vi "Motor_Lumicks_Meng.vi"() -> ()   [LabVIEW 2014]
uses:
  <vilib>/userdefined/High Color/IMAQdx.ctl
  <vilib>/Utility/inputDevices.llb/joystickAcquire.vi
  <vilib>/Utility/inputDevices.llb/closeJoystick.vi
  <vilib>/vision/driver/NI_Vision_Acquisition_Software.lvlib
panel:
  out "error out 2":errorcluster
  out "Image":T1(plugin-control)
  in  "Goto Channel 5":bool
  in  "Goto Channel 4":bool
  in  "Capture Channel 5":bool
  in  "Capture Channel 4":bool
  out "Channel 5":T2={"X Pos (mm)"=0.00014575559, "Y Pos (mm)"=-0.0013701026, "Z Pos (mm)"=0.004635028} {"Y Pos (mm)" format="%.3f"; "Z Pos (mm)" format="%.3f"; "X Pos (mm)" format="%.3f"}
  out "Channel 4":T2={"X Pos (mm)"=0.00014575559, "Y Pos (mm)"=-0.0013701026, "Z Pos (mm)"=0.004635028} {"Y Pos (mm)" format="%.3f"; "Z Pos (mm)" format="%.3f"; "X Pos (mm)" format="%.3f"}
  in  "Stop All":bool=TRUE
  out "button 4":bool
  in  "button 3":bool
  in  "Motor Cruise Param":T3={"X Acc (mm/s^2)"=0.1, "X Vmax (mm/s)"=1.0, "Y Acc (mm/s^2)"=0.3, "Y Vmax (mm/s)"=1.0, "Z Acc (mm/s^2)"=0.1, "Z Vmax (mm/s)"=0.1}
  out "XYZ position":sgl[](array[numeric])=[1.7793261, 1.7925023, 3.857043]
  in  "Motor Limits":T4={"XMAX"=12.0, "XMIN"=-12.0, "YMAX"=12.0, "YMIN"=-12.0, "ZMAX"=10.0, "ZMIN"=-10.0}
  in  "Motor settings (X,Y)":cluster{"Vmax (mm/s)":sgl, "Acc (mm/s/s)":sgl}={"Vmax (mm/s)"=0.05, "Acc (mm/s/s)"=0.2}
  in  "Motor settings (Z)":cluster{"Vmax (mm/s)":sgl, "Acc (mm/s/s)":sgl}={"Vmax (mm/s)"=0.02, "Acc (mm/s/s)"=0.2}
  in  "Capture Channel 3":bool
  in  "Capture Channel 2":bool
  in  "Capture Channel 1":bool
  in  "Goto Channel 2":bool
  in  "Goto Channel 3":bool
  in  "Goto Channel 1":bool
  out "Channel 1":T2={"X Pos (mm)"=2.683244, "Y Pos (mm)"=-0.037109375, "Z Pos (mm)"=0.2016383} {"Y Pos (mm)" format="%.3f"; "Z Pos (mm)" format="%.3f"; "X Pos (mm)" format="%.3f"}
  out "Channel 2":T2={"X Pos (mm)"=2.3714144, "Y Pos (mm)"=-0.4775245, "Z Pos (mm)"=0.20615672} {"Y Pos (mm)" format="%.3f"; "Z Pos (mm)" format="%.3f"; "X Pos (mm)" format="%.3f"}
  out "Channel 3":T2={"X Pos (mm)"=3.6928055, "Y Pos (mm)"=-0.788188, "Z Pos (mm)"=0.19962686} {"Y Pos (mm)" format="%.3f"; "Z Pos (mm)" format="%.3f"; "X Pos (mm)" format="%.3f"}
  out "error out":errorcluster
  in  "MG17Motor Z":refnum<k7>(container)
  in  "MG17Motor Y":refnum<k7>(container)
  in  "MG17Motor X":refnum<k7>(container)
  out "Stage Moving":bool
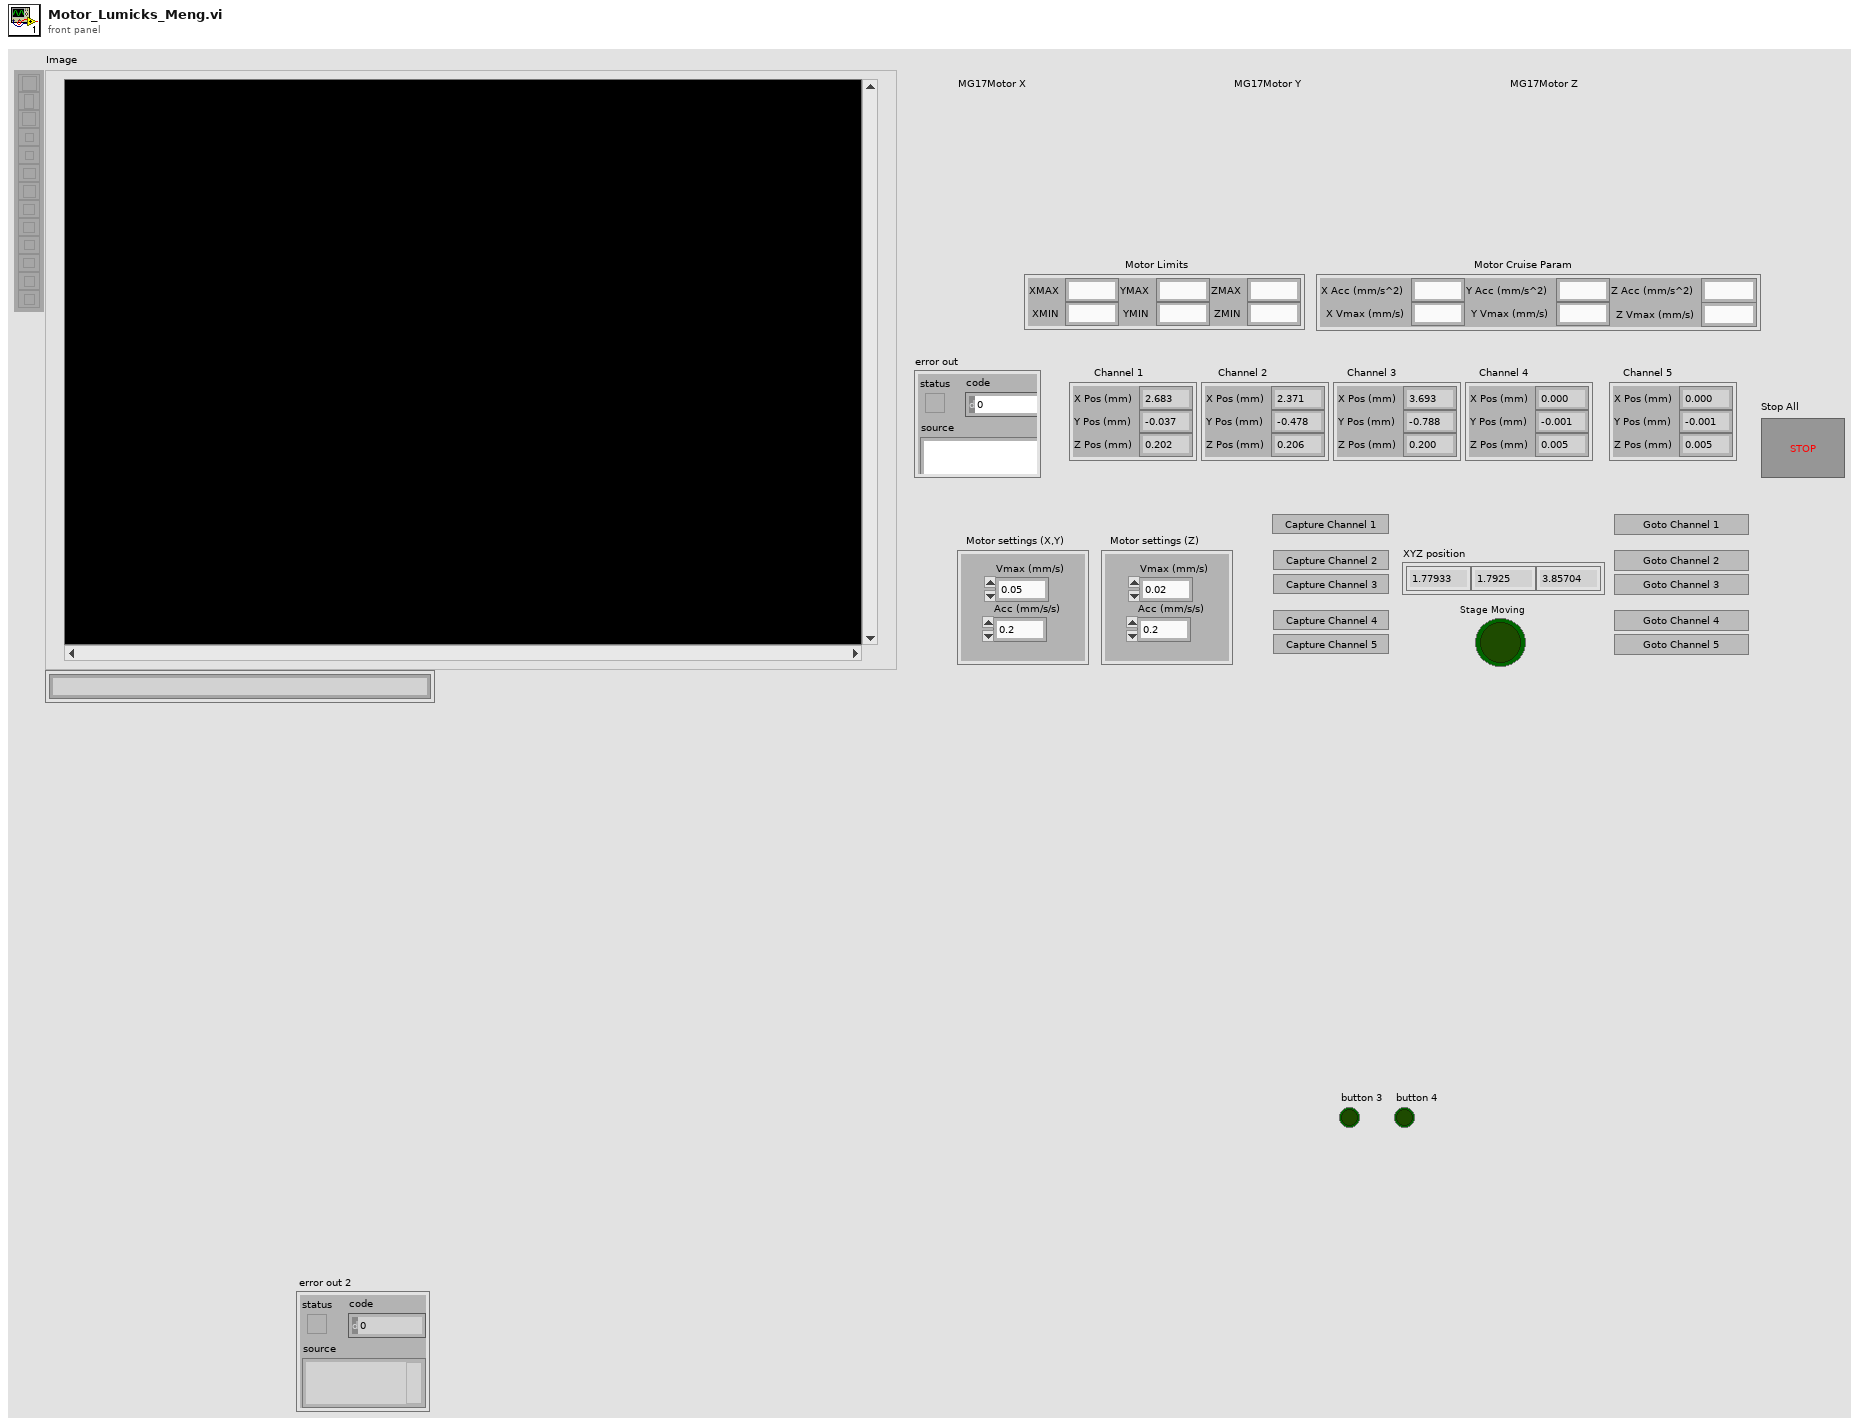
[diagram p1: front panel]
types:
  T1 = typedef "IMAQ Image.ctl" = refnum<image>
  T2 = cluster{"X Pos (mm)":sgl, "Y Pos (mm)":sgl, "Z Pos (mm)":sgl}
  T3 = cluster{"X Acc (mm/s^2)":sgl, "X Vmax (mm/s)":sgl, "Y Acc (mm/s^2)":sgl, "Y Vmax (mm/s)":sgl, "Z Acc (mm/s^2)":sgl, "Z Vmax (mm/s)":sgl}
  T4 = cluster{"XMAX":sgl, "XMIN":sgl, "YMAX":sgl, "YMIN":sgl, "ZMAX":sgl, "ZMIN":sgl}
  T5 = typedef "IMAQdx.ctl" = refnum<k21>
  T6 = typedef "Image Type" = u32
  T7 = cluster{"X axis":i32, "Y axis":i32, "Z axis":i32, "X axis rotation":i32, "Y axis rotation":i32, "Z axis rotation":i32, "U axis":i32, "V axis":i32}
  T8 = cluster{"button 1":bool, "button 2":bool, "button 3":bool, "button 4":bool, "button 5":bool, "button 6":bool, "button 7":bool, "button 8":bool, "button 9":bool, "button 10":bool, "button 11":bool, "button 12":bool, "button 13":bool, "button 14":bool, "button 15":bool, "button 16":bool, "button 17":bool, "button 18":bool, "button 19":bool, "button 20":bool, "button 21":bool, "button 22":bool, "button 23":bool, "button 24":bool, "button 25":bool, "button 26":bool, "button 27":bool, "button 28":bool, "button 29":bool, "button 30":bool, "button 31":bool, "button 32":bool}
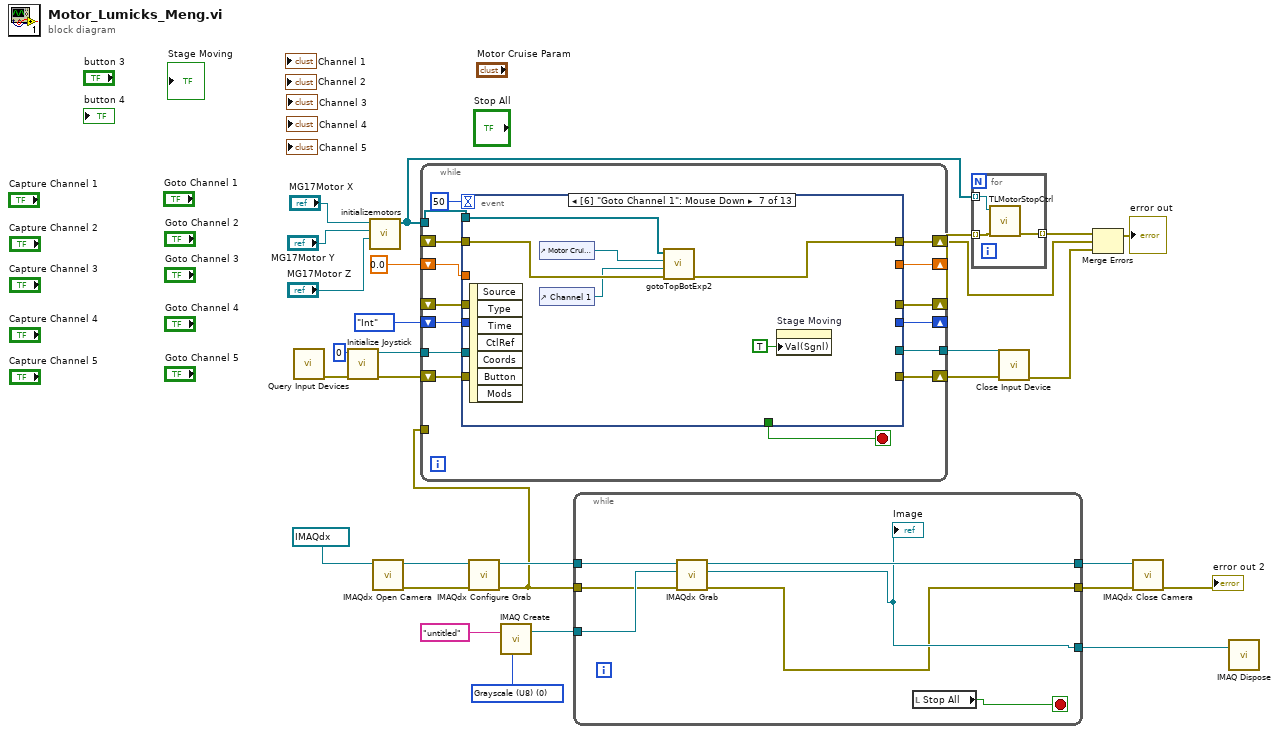
[diagram p0: block diagram]
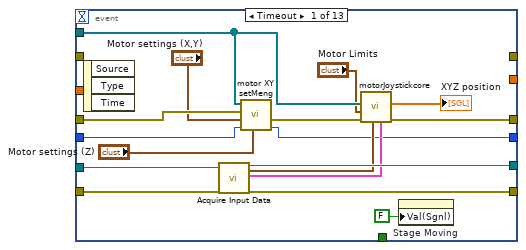
[diagram p2: hidden frame]
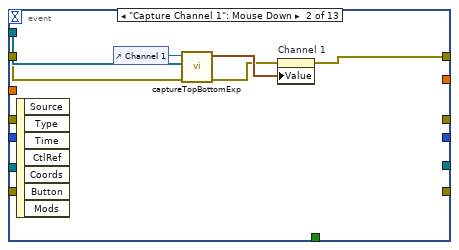
[diagram p3: hidden frame]
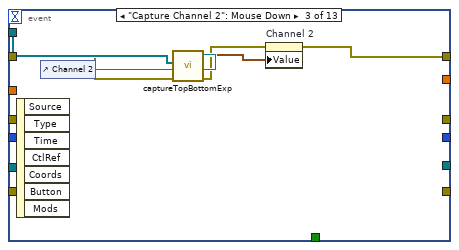
[diagram p4: hidden frame]
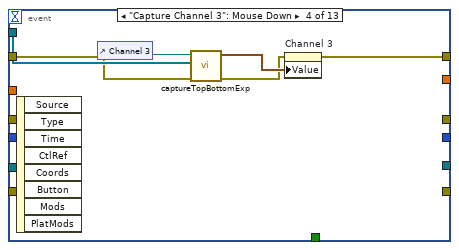
[diagram p5: hidden frame]
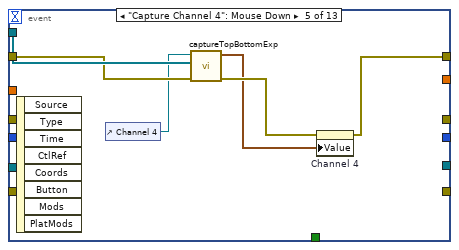
[diagram p6: hidden frame]
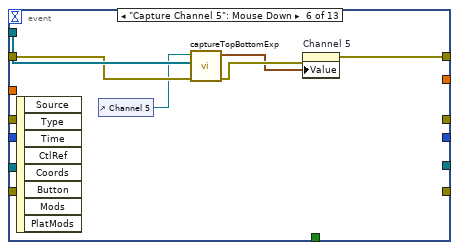
[diagram p7: hidden frame]
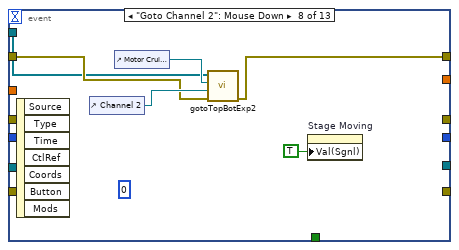
[diagram p8: hidden frame]
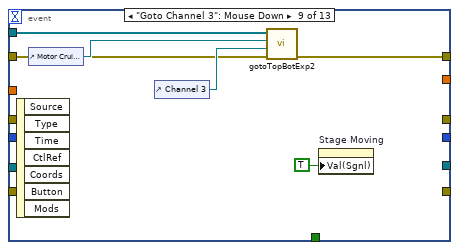
[diagram p9: hidden frame]
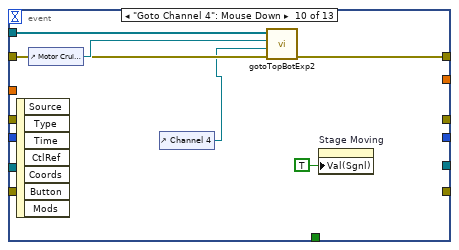
[diagram p10: hidden frame]
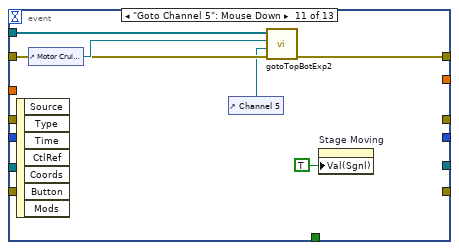
[diagram p11: hidden frame]
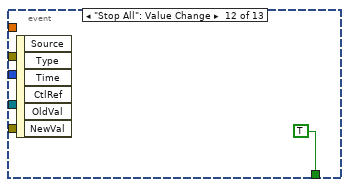
[diagram p12: hidden frame]
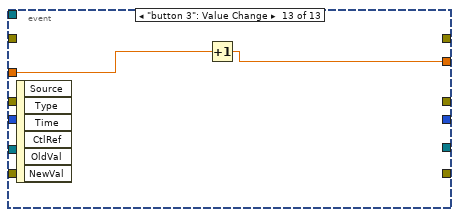
[diagram p13: hidden frame]
diagram:
  w6 = T6 0 items=["Grayscale (U8)", "Grayscale (I16)", "Grayscale (SGL)", "Complex (CSG)", "RGB (U32)", "HSL (U32)", "RGB (U64)", "Grayscale (U16)"] ("Image Type")
  n1 = call <vilib>:"Query Input Devices.vi"() -> ("error out"=w22:errorcluster)  [unwired: 8 in, 3 out]
  n2 = call <vilib>:"Initialize Joystick.vi"("error in (no error)"=w22, "device index"=0) -> ("error out"=w19:errorcluster, "device ID"=w20:refnum<k1>)  [unwired: 8 in]
  n3 = call "initializemotors.vi"("MG17Motor Z"="MG17Motor Z", "MG17Motor Y"="MG17Motor Y", "Automation Refnum in"="MG17Motor X") -> ("Array 2"=w24:refnum<k7>[])  [unwired: 7 in, 1 out]
  n4 = call <vilib>:"IMAQdx Open Camera.vi"("Session In"=T5 "cam0") -> ("error out"=w10:errorcluster, "Session Out"=w9:T5)  [unwired: 9 in]
  n5 = call <vilib>:"IMAQdx Configure Grab.vi"("error in"=w10, "Session In"=w9) -> ("error out"=w1:errorcluster, "Session Out"=w8:T5)  [unwired: 8 in]
  n6 = while {
    tunnel: w24 -> [w44]
    shift-right: [w43] -> w14
    shift-left: _ -> [w42]
    shift-right: [w39] -> _
    shift-left: 0.0 -> [w40]
    tunnel: w20 -> [w38]
    shift-right: [w36] -> w18
    shift-left: w19 -> [w37]
    tunnel: [w35] -> w17
    shift-right: [w34] -> w15
    shift-left: _ -> [w33]
    shift-right: [w31] -> _
    shift-left: enum16{"Int", "Set"}."Int" ("Enum") -> [w32]
    tunnel: w1 -> [_]
    stop <- w41 stop-if-true
    n7 = event shown="[6] \"Goto Channel 1\": Mouse Down" {
      selector: _ -> [_ _ _ _ _ _ _ _ _ _ _ _ _]
      dyn-events: _ -> [_ _ _ _ _ _ _ _ _ _ _ _ _]
      timeout: 50 -> [_ _ _ _ _ _ _ _ _ _ _ _ _]
      tunnel: w44 -> [w51 w67 w72 w79 w85 w91 w93 w99 w105 w112 w118 _ _]
      tunnel: [_ w64 w68 w74 w81 w86 w96 w100 w106 w113 w119 _ _] -> w43
      tunnel: w42 -> [_ w63 w71 w77 w84 w90 w97 w101 w107 w114 w120 _ _]
      tunnel: [_ _ _ _ _ _ _ _ _ _ _ TRUE _] -> w41
      tunnel: [_ _ _ _ _ _ _ _ _ _ _ _ w124] -> w39
      tunnel: w40 -> [_ _ _ _ _ _ _ _ _ _ _ _ w123]
      tunnel: w38 -> [w61 _ _ _ _ _ _ _ _ _ _ _ _]
      tunnel: w37 -> [w60 _ _ _ _ _ _ _ _ _ _ _ _]
      tunnel: [w59 _ _ _ _ _ _ _ _ _ _ _ _] -> w36
      tunnel: [w58 _ _ _ _ _ _ _ _ _ _ _ _] -> w35
      tunnel: [w54 _ _ _ _ _ _ _ _ _ _ _ _] -> w34
      tunnel: w33 -> [w53 _ _ _ _ _ _ _ _ _ _ _ _]
      tunnel: w32 -> [w47 _ _ _ _ _ _ _ _ _ _ _ _]
      tunnel: [w46 _ _ _ _ _ _ _ _ _ _ _ _] -> w31
      event Timeout {
        n8 = event-data() -> ()  [unwired: 1 in, 3 out]
        n9 = call-poly <vilib>:"Acquire Input Data.vi"("device ID"=w61, "error in (no error)"=w60) -> ("device ID"=w58:refnum<k1>, "axis info"=w56:T7, "button info"=w57:T8, "error out"=w59:errorcluster)  [unwired: 13 in, 1 out]
        n10 = call "motor XY setMeng.vi"("Motor settings Z"="Motor settings (Z)", "Enum in"=w47, "Motor settings (X,Y)"="Motor settings (X,Y)", "Array"=w53, "Array 2"=w51) -> ("Enum out"=w46:enum16{"Int", "Set"}, "Array 3"=w52:errorcluster[])  [unwired: 4 in, 1 out]
        n11 = call "motorJoystickcore.vi"("button info"=w57, "axis info"=w56, "error in"=w52, "Motor Limits"="Motor Limits", "Array in"=w51) -> ("error out"=w54:errorcluster[], "XYZ position"=→"XYZ position":sgl[])  [unwired: 5 in]
        n12 = property on="Stage Moving" class="Bool (strict)"("Val(Sgnl)"=FALSE ("Value (Signaling)")) -> ()  [unwired: 2 in, 2 out]
      }
      event "Capture Channel 1": Mouse Down {
        n13 = event-data() -> ()  [unwired: 1 in, 7 out]
        n14 = control-ref of="Channel 1"() -> (w62:refnum<vi>)
        n15 = call "captureTopBottomExp.vi"("error in (no error)"=w63, "Array in"=w67, "Cluster in"=w62) -> ("error out"=w65:errorcluster, "Value"=w66:T2)  [unwired: 7 in]
        n16 = property on="Channel 1" class="Clust (strict)"(error in=w65, "Value"=w66) -> (error out=w64:errorcluster)  [unwired: 1 in, 1 out]
      }
      event "Capture Channel 2": Mouse Down {
        n17 = event-data() -> ()  [unwired: 1 in, 7 out]
        n18 = control-ref of="Channel 2"() -> (w73:refnum<vi>)
        n19 = call "captureTopBottomExp.vi"("error in (no error)"=w71, "Array in"=w72, "Cluster in"=w73) -> ("error out"=w69:errorcluster, "Value"=w70:T2)  [unwired: 7 in]
        n20 = property on="Channel 2" class="Clust (strict)"(error in=w69, "Value"=w70) -> (error out=w68:errorcluster)  [unwired: 1 in, 1 out]
      }
      event "Capture Channel 3": Mouse Down {
        n21 = event-data() -> ()  [unwired: 1 in, 8 out]
        n22 = control-ref of="Channel 3"() -> (w78:refnum<vi>)
        n23 = call "captureTopBottomExp.vi"("error in (no error)"=w77, "Array in"=w79, "Cluster in"=w78) -> ("error out"=w75:errorcluster, "Value"=w76:T2)  [unwired: 7 in]
        n24 = property on="Channel 3" class="Clust (strict)"(error in=w75, "Value"=w76) -> (error out=w74:errorcluster)  [unwired: 1 in, 1 out]
      }
      event "Capture Channel 4": Mouse Down {
        n25 = event-data() -> ()  [unwired: 1 in, 8 out]
        n26 = control-ref of="Channel 4"() -> (w83:refnum<vi>)
        n27 = call "captureTopBottomExp.vi"("error in (no error)"=w84, "Array in"=w85, "Cluster in"=w83) -> ("error out"=w82:errorcluster, "Value"=w80:T2)  [unwired: 7 in]
        n28 = property on="Channel 4" class="Clust (strict)"(error in=w82, "Value"=w80) -> (error out=w81:errorcluster)  [unwired: 1 in, 1 out]
      }
      event "Capture Channel 5": Mouse Down {
        n29 = event-data() -> ()  [unwired: 1 in, 8 out]
        n30 = control-ref of="Channel 5"() -> (w89:refnum<vi>)
        n31 = call "captureTopBottomExp.vi"("error in (no error)"=w90, "Array in"=w91, "Cluster in"=w89) -> ("error out"=w88:errorcluster, "Value"=w87:T2)  [unwired: 7 in]
        n32 = property on="Channel 5" class="Clust (strict)"(error in=w88, "Value"=w87) -> (error out=w86:errorcluster)  [unwired: 1 in, 1 out]
      }
      event "Goto Channel 1": Mouse Down {
        n33 = event-data() -> ()  [unwired: 1 in, 7 out]
        n34 = control-ref of="Motor Cruise Param"() -> (w95:refnum<vi>)
        n35 = control-ref of="Channel 1"() -> (w94:refnum<vi>)
        n36 = call "gotoTopBotExp2.vi"("error in (no error)"=w97, "position"=w94, "motor setting"=w95, "appended array"=w93) -> ("error out"=w96:errorcluster)  [unwired: 7 in]
        n37 = property on="Stage Moving" class="Bool (strict)"("Val(Sgnl)"=TRUE ("Value (Signaling)")) -> ()  [unwired: 2 in, 2 out]
      }
      event "Goto Channel 2": Mouse Down {
        (unwired) 0 ("lChanID")
        n38 = event-data() -> ()  [unwired: 1 in, 7 out]
        n39 = control-ref of="Channel 2"() -> (w102:refnum<vi>)
        n40 = control-ref of="Motor Cruise Param"() -> (w103:refnum<vi>)
        n41 = call "gotoTopBotExp2.vi"("error in (no error)"=w101, "position"=w102, "motor setting"=w103, "appended array"=w99) -> ("error out"=w100:errorcluster)  [unwired: 7 in]
        n42 = property on="Stage Moving" class="Bool (strict)"("Val(Sgnl)"=TRUE ("Value (Signaling)")) -> ()  [unwired: 2 in, 2 out]
      }
      event "Goto Channel 3": Mouse Down {
        n43 = event-data() -> ()  [unwired: 1 in, 7 out]
        n44 = control-ref of="Motor Cruise Param"() -> (w109:refnum<vi>)
        n45 = control-ref of="Channel 3"() -> (w108:refnum<vi>)
        n46 = call "gotoTopBotExp2.vi"("error in (no error)"=w107, "position"=w108, "motor setting"=w109, "appended array"=w105) -> ("error out"=w106:errorcluster)  [unwired: 7 in]
        n47 = property on="Stage Moving" class="Bool (strict)"("Val(Sgnl)"=TRUE ("Value (Signaling)")) -> ()  [unwired: 2 in, 2 out]
      }
      event "Goto Channel 4": Mouse Down {
        n48 = event-data() -> ()  [unwired: 1 in, 7 out]
        n49 = control-ref of="Motor Cruise Param"() -> (w115:refnum<vi>)
        n50 = control-ref of="Channel 4"() -> (w110:refnum<vi>)
        n51 = call "gotoTopBotExp2.vi"("error in (no error)"=w114, "position"=w110, "motor setting"=w115, "appended array"=w112) -> ("error out"=w113:errorcluster)  [unwired: 7 in]
        n52 = property on="Stage Moving" class="Bool (strict)"("Val(Sgnl)"=TRUE ("Value (Signaling)")) -> ()  [unwired: 2 in, 2 out]
      }
      event "Goto Channel 5": Mouse Down {
        n53 = event-data() -> ()  [unwired: 1 in, 7 out]
        n54 = control-ref of="Motor Cruise Param"() -> (w121:refnum<vi>)
        n55 = control-ref of="Channel 5"() -> (w116:refnum<vi>)
        n56 = call "gotoTopBotExp2.vi"("error in (no error)"=w120, "position"=w116, "motor setting"=w121, "appended array"=w118) -> ("error out"=w119:errorcluster)  [unwired: 7 in]
        n57 = property on="Stage Moving" class="Bool (strict)"("Val(Sgnl)"=TRUE ("Value (Signaling)")) -> ()  [unwired: 2 in, 2 out]
      }
      event "Stop All": Value Change {
        n58 = event-data() -> ()  [unwired: 1 in, 6 out]
      }
      event "button 3": Value Change {
        n59 = event-data() -> ()  [unwired: 1 in, 6 out]
        n60 = Increment(x=w123) -> (x+1=w124:dbl)
      }
    }
  }
  n61 = call "IMAQ Create"("Image Name"="untitled", "Image Type"=w6) -> ("New Image"=w12:T1)  [unwired: 3 in, 1 out]
  n62 = while {
    tunnel: w12 -> [w130]
    tunnel: w8 -> [w131]
    tunnel: w1 -> [w129]
    tunnel: [w125] -> w5
    tunnel: [w128] -> w4
    tunnel: [w126] -> w2
    stop <- w127 stop-if-true
    n63 = call <vilib>:"IMAQdx Grab.vi"("error in"=w129, "Image In"=w130, "Session In"=w131) -> ("error out"=w125:errorcluster, "Image Out"=w126:T1, "Session Out"=w128:T5)  [unwired: 5 in, 1 out]
    "Image" <- w126
    n64 = local read "Stop All"() -> (w127:bool)
  }
  n65 = for {
    tunnel: w24 -> [w134] mode=indexing
    tunnel: w15 -> [w133] mode=indexing
    tunnel: [w132] -> w26 mode=indexing
    n66 = call "TLMotorStopCtrl.vi"("Error In (No Error)"=w133, "Motor Ref"=w134) -> ("Error Out"=w132:errorcluster)  [unwired: 4 in, 1 out]
  }
  n67 = call-poly <vilib>:"Close Input Device.vi"("error in (no error)"=w18, "device ID"=w17) -> ("error out"=w13:errorcluster)  [unwired: 8 in]
  n68 = Merge Errors(w26, w14, w13) -> (→"error out":errorcluster)
  n69 = call <vilib>:"IMAQdx Close Camera.vi"("error in"=w5, "Session In"=w4) -> ("error out"=→"error out 2":errorcluster)  [unwired: 9 in]
  n70 = call "IMAQ Dispose"("Image"=w2) -> ()  [unwired: 5 in, 1 out]
